vi "Check data and buffor size (SubVI).vi"(10 "data size":i32, 11 "Analog output in":refnum<class "Analog output.lvclass">) -> (0 "Error message":string="Analog output write.\n\nNumber of samples in data must be the same as Buffor size\nconfigured in Create channel/Configure channel.", 1 "Error?":bool)   [LabVIEW 2009, in "MicroDAQ.lvlib" / "Analog output.lvclass"]
uses:
  <instrlib>/MicroDAQ/Channel/Analog Output/Analog output.lvclass
  <instrlib>/MicroDAQ/Channel/Analog Output/Analog output.lvclass/Analog output.ctl
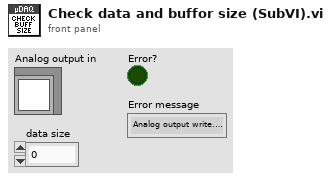
[diagram p1: front panel]
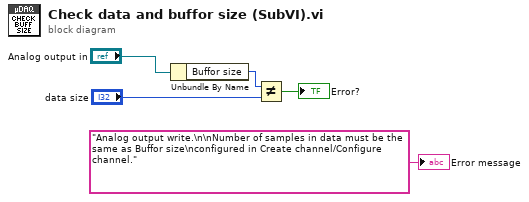
[diagram p0: block diagram]
diagram:
  n1 = Unbundle By Name("Analog output in") -> ("Buffor size"=w5:i32)
  n2 = Not Equal?(x=w5, y="data size") -> (x != y?=→"Error?":bool)
  "Error message" <- "Analog output write.\n\nNumber of samples in data must be the same as Buffor size\nconfigured in Create channel/Configure channel."
